vi "Update MulticolumnListbox.vi"(10 "frame map":map{string, T1}(c390), 11 "Frames 2":refnum<vi>) -> ()   [LabVIEW 2020]
uses:
  <instrlib>/AIM GmbH/_AIM 664/_controls/queue_header_generic.ctl
  <instrlib>/AIM GmbH/_AIM 664/AIM664LV.lvlib
  controls/frame_record_type.ctl
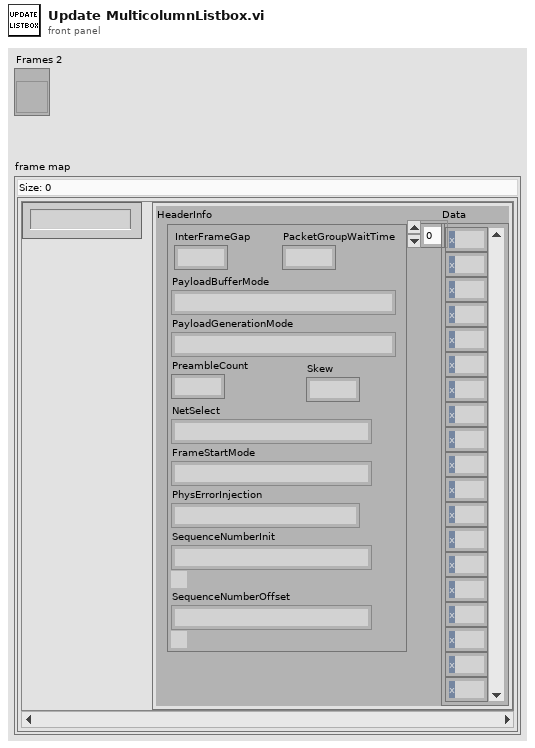
[diagram p1: front panel]
types:
  T1 = typedef "frame_record_type.ctl" = cluster{"HeaderInfo":T2, "Data":u8[]}
  T2 = typedef "AIM664LV.lvlib/queue_header_generic.ctl" = cluster{"InterFrameGap":u32, "PacketGroupWaitTime":u32, "PayloadBufferMode":u8, "PayloadGenerationMode":u8, "PreambleCount":u8, "Skew":u32, "NetSelect":u8, "FrameStartMode":u8, "PhysErrorInjection":u32, "SequenceNumberInit":u16, "SequenceNumberOffset":u16}
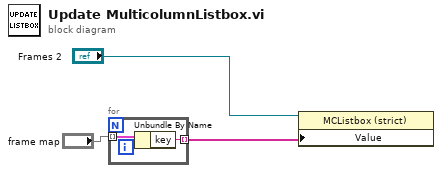
[diagram p0: block diagram]
diagram:
  n1 = for {
    tunnel: "frame map" -> [w5] mode=indexing
    tunnel: [w4] -> w2 mode=indexing
    n2 = Unbundle By Name(w5) -> ("key"=w4:string)
  }
  n3 = property on="Property Node" class="MCListbox (strict)"(reference="Frames 2", "Value"=w2) -> ()  [unwired: 1 in, 2 out]
